vi "endeff-GS-comm.vi"() -> ()   [LabVIEW 2016]
panel:
  out "left":dbl
  in  "Select command to send:":string(combo)
  out "tOp":dbl
  out "Tilt":dbl
  out "Full Data String from Ethernet":string
  in  "Start":bool
  out "Pan":dbl
  out "Right":dbl
  in  "Stop":bool
  # "End effector - Ground Station \ncommunication interface"
  # "DISTANCE SENSORS:"
  # "PAN AND TILT MOTORS:"
  # "mm"
  # "deg"
  # "mm"
  # "deg"
  # "mm"
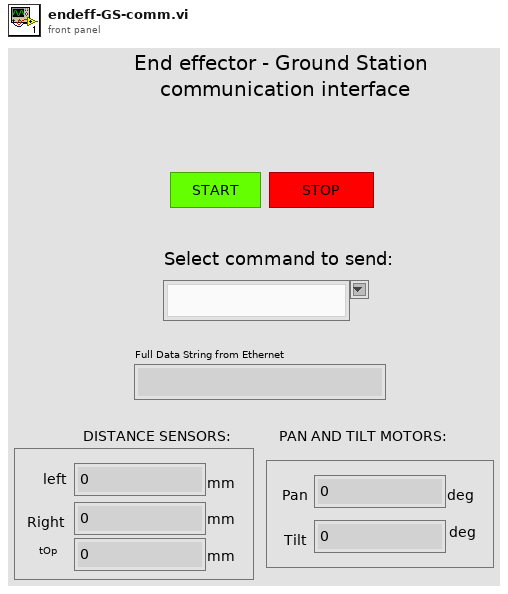
[diagram p1: front panel]
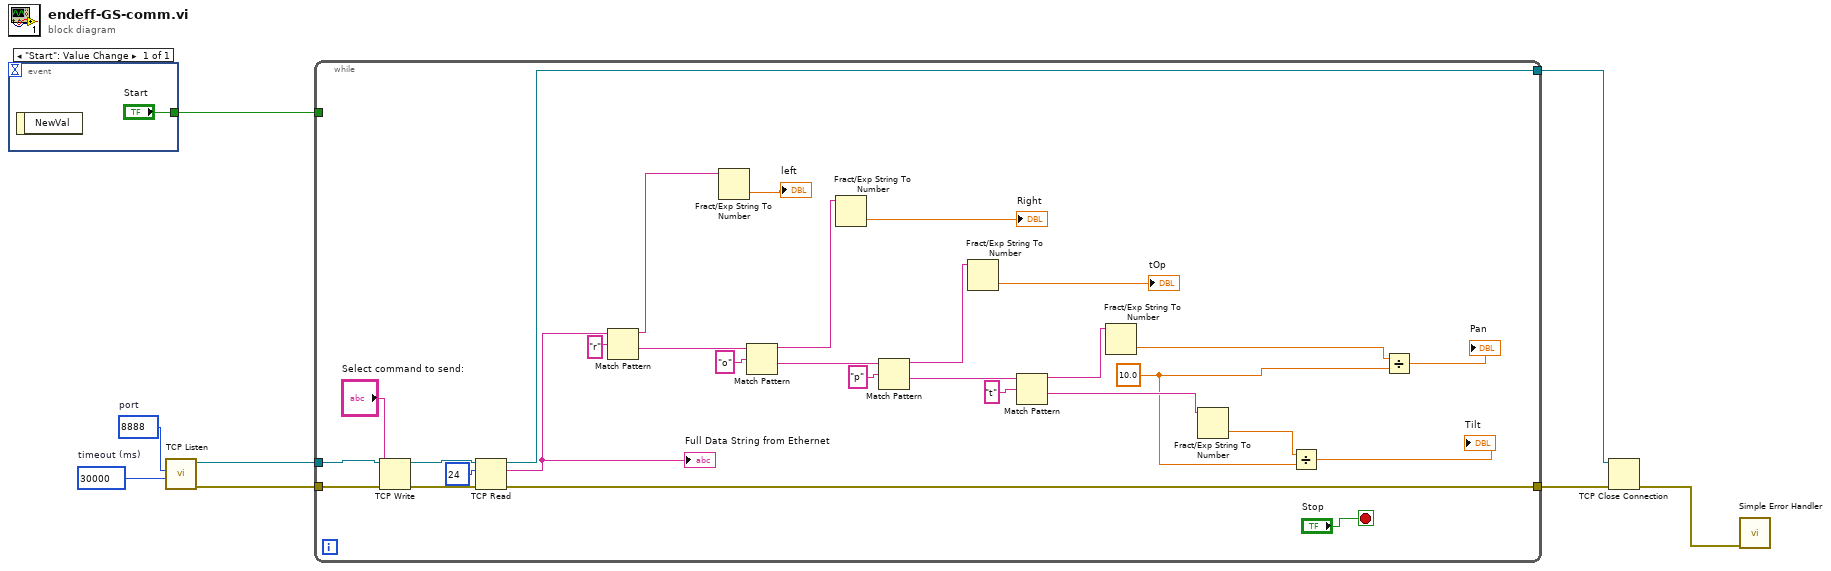
[diagram p0: block diagram]
diagram:
  w7 = u16 8888  # port
  w8 = 30000  # timeout (ms)
  n1 = event shown="[0] \"Start\": Value Change" {
    selector: _ -> [_]
    dyn-events: _ -> [_]
    timeout: _ -> [_]
    tunnel: ["Start"] -> w1
    event "Start": Value Change {
      n2 = event-data() -> ()  [unwired: 1 in, 1 out]
    }
  }
  n3 = call <vilib>:"TCP Listen.vi"("timeout ms (wait forever: -1)"=w8, "port"=w7) -> ("error out"=w4:errorcluster, "connection ID"=w5:refnum<k5>)  [unwired: 5 in, 3 out]
  n4 = while {
    tunnel: w5 -> [w28]
    tunnel: w4 -> [w27]
    tunnel: [w24] -> w3
    tunnel: [w23] -> w2
    tunnel: w1 -> [_]
    stop <- "Stop" stop-if-true
    w11 = 10.0 ("y")
    n5 = TCP Write(connection ID=w28, data in="Select command to send:", error in (no error)=w27) -> (connection ID out=w25:refnum<k5>, error out=w26:errorcluster)  [unwired: 1 in, 1 out]
    n6 = TCP Read(connection ID=w25, bytes to read=24, error in (no error)=w26) -> (connection ID out=w24:refnum<k5>, data out=w22:string, error out=w23:errorcluster)  [unwired: 2 in]
    "Full Data String from Ethernet" <- w22
    n7 = Match Pattern(string=w22, regular expression="r") -> (before substring=w17:string, after substring=w38:string)  [unwired: 1 in, 2 out]
    n8 = Fract/Exp String To Number(string=w17) -> (number=→"left":dbl)  [unwired: 3 in, 1 out]
    n9 = Match Pattern(string=w38, regular expression="o") -> (before substring=w33:string, after substring=w37:string)  [unwired: 1 in, 2 out]
    n10 = Fract/Exp String To Number(string=w33) -> (number=→"Right":dbl)  [unwired: 3 in, 1 out]
    n11 = Match Pattern(string=w37, regular expression="p") -> (before substring=w20:string, after substring=w31:string)  [unwired: 1 in, 2 out]
    n12 = Fract/Exp String To Number(string=w20) -> (number=→"tOp":dbl)  [unwired: 3 in, 1 out]
    n13 = Match Pattern(string=w31, regular expression="t") -> (before substring=w30:string, after substring=w18:string)  [unwired: 1 in, 2 out]
    n14 = Fract/Exp String To Number(string=w30) -> (number=w15:dbl)  [unwired: 3 in, 1 out]
    n15 = Fract/Exp String To Number(string=w18) -> (number=w14:dbl)  [unwired: 3 in, 1 out]
    n16 = Divide(x=w14, y=w11) -> (x/y=→"Tilt":dbl)
    n17 = Divide(x=w15, y=w11) -> (x/y=→"Pan":dbl)
  }
  n18 = TCP Close Connection(connection ID=w3, error in (no error)=w2) -> (error out=w6:errorcluster)  [unwired: 1 in, 1 out]
  n19 = call <vilib>:"Simple Error Handler.vi"("error in (no error)"=w6) -> ()  [unwired: 4 in, 5 out]
